vi "VALEW_ATC_Non-concurrent Verify Valve Timing.vi"(0 "High Times (s)":dbl[][](array[numeric])=[[0.048, 19.932000000000002, 0.0], [0.256, 9.626, 10.098], [0.254, 9.628, 10.098], [0.256, 9.625, 10.099], [0.047, 19.933, 0.0], [0.253, 10.701, 9.026], [0.255, 10.699, 9.026], [0.048, 19.932000000000002, 0.0], [0.258, 8.014, 11.708], [0.256, 8.016, 11.708], [0.256, 8.016, 11.708], [0.048, 19.932000000000002, 0.0], [0.254, 7.527, 12.199], [0.047, 19.933, 0.0], [0.253, 6.848, 12.879]], 7 "Total cold ON time (s)":dbl, 11 "Total hot ON time (s)":dbl) -> (6 "Pass/Fail?":bool, 10 "Report Text":string)   [LabVIEW 2016, in "TLMB.lvlib"]
uses:
  Projects/TLMB.lvlib
panel:
  # "off"
  # "on"
  # "off"
  # "on"
  # "off"
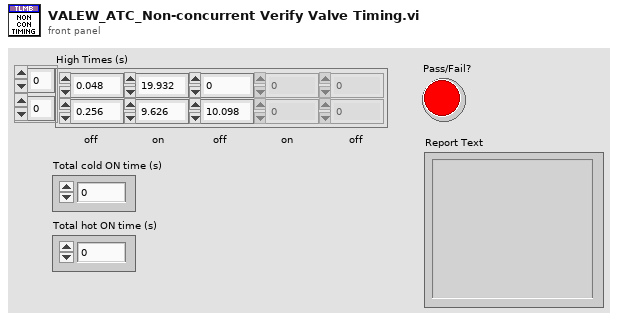
[diagram p1: front panel]
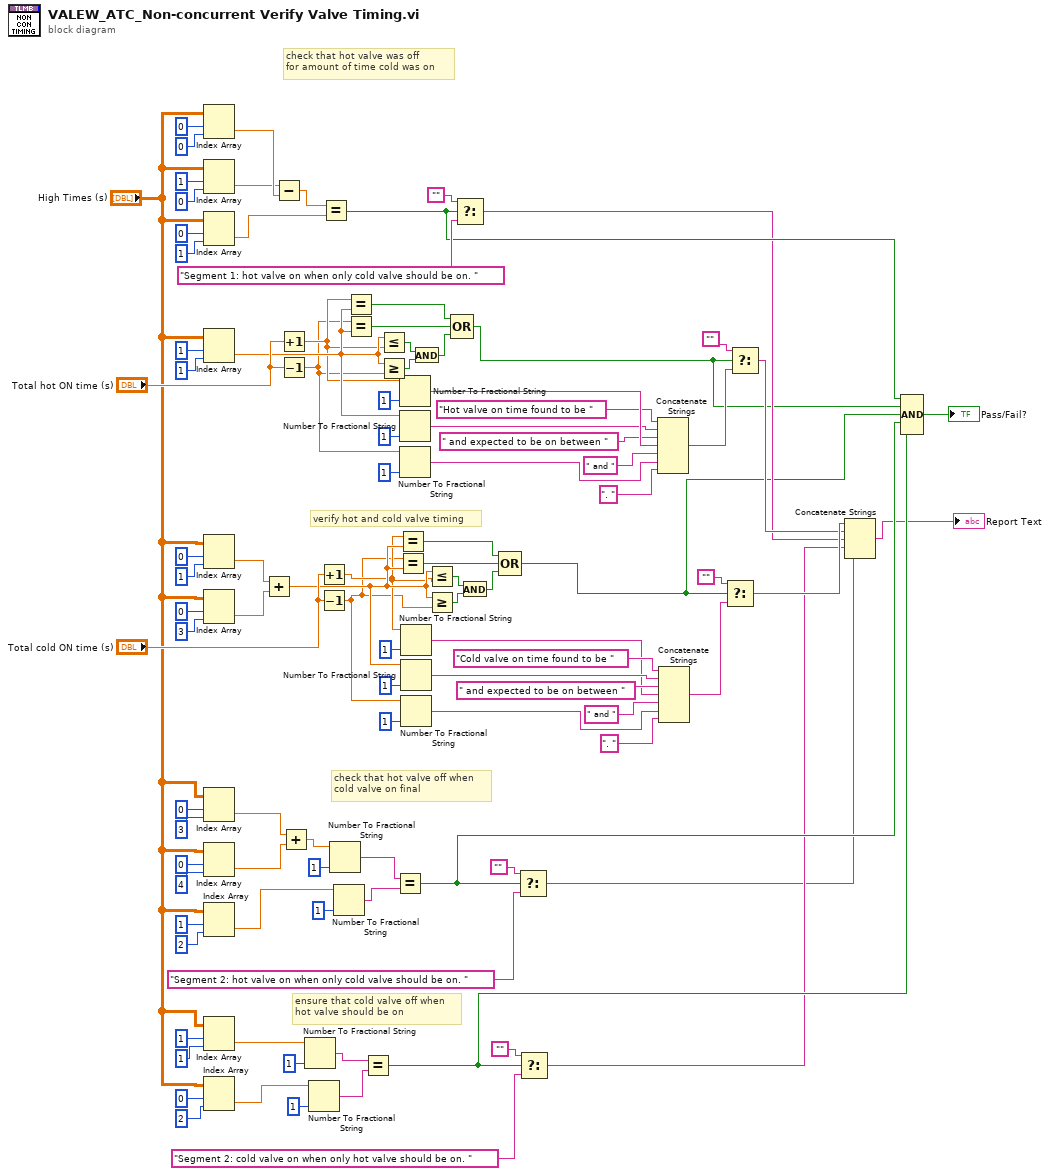
[diagram p0: block diagram]
diagram:
  # "verify hot and cold valve timing"
  # "ensure that cold valve off when\nhot valve should be on"
  # "check that hot valve off when\ncold valve on final"
  # "check that hot valve was off\nfor amount of time cold was on"
  n1 = Index Array(array="High Times (s)", index (row)=0, index (col)=0 ("disabled index (col)")) -> (element=w34:dbl)
  n2 = Index Array(array="High Times (s)", index (row)=1, index (col)=0 ("disabled index (col)")) -> (element=w33:dbl)
  n3 = Index Array(array="High Times (s)", index (row)=0, index (col)=1 ("disabled index (col)")) -> (element=w99:dbl)
  n4 = Index Array(array="High Times (s)", index (row)=1, index (col)=1 ("disabled index (col)")) -> (element=w15:dbl)
  n5 = Index Array(array="High Times (s)", index (row)=0, index (col)=1 ("disabled index (col)")) -> (element=w88:dbl)
  n6 = Index Array(array="High Times (s)", index (row)=0, index (col)=3 ("disabled index (col)")) -> (element=w89:dbl)
  n7 = Index Array(array="High Times (s)", index (row)=0, index (col)=3 ("disabled index (col)")) -> (element=w80:dbl)
  n8 = Index Array(array="High Times (s)", index (row)=0, index (col)=4 ("disabled index (col)")) -> (element=w79:dbl)
  n9 = Index Array(array="High Times (s)", index (row)=1, index (col)=2 ("disabled index (col)")) -> (element=w7:dbl)
  n10 = Index Array(array="High Times (s)", index (row)=1, index (col)=1 ("disabled index (col)")) -> (element=w1:dbl)
  n11 = Index Array(array="High Times (s)", index (row)=0, index (col)=2 ("disabled index (col)")) -> (element=w2:dbl)
  n12 = Add(x=w88, y=w89) -> (x+y=w21:dbl)
  n13 = Subtract(x=w33, y=w34) -> (x-y=w32:dbl)
  n14 = Increment(x="Total hot ON time (s)") -> (x+1=w14:dbl)
  n15 = Decrement(x="Total hot ON time (s)") -> (x-1=w13:dbl)
  n16 = Add(x=w80, y=w79) -> (x+y=w9:dbl)
  n17 = Number To Fractional String(number=w1, precision (6)=i16 1) -> (F-format string=w4:string)  [unwired: 2 in]
  n18 = Number To Fractional String(number=w2, precision (6)=i16 1) -> (F-format string=w3:string)  [unwired: 2 in]
  n19 = Increment(x="Total cold ON time (s)") -> (x+1=w20:dbl)
  n20 = Decrement(x="Total cold ON time (s)") -> (x-1=w19:dbl)
  n21 = Equal?(x=w32, y=w99) -> (x = y?=w46:bool)
  n22 = Number To Fractional String(number=w9, precision (6)=i16 1) -> (F-format string=w8:string)  [unwired: 2 in]
  n23 = Number To Fractional String(number=w7, precision (6)=i16 1) -> (F-format string=w11:string)  [unwired: 2 in]
  n24 = Equal?(x=w14, y=w15) -> (x = y?=w27:bool)
  n25 = Equal?(x=w13, y=w15) -> (x = y?=w26:bool)
  n26 = Equal?(x=w4, y=w3) -> (x = y?=w43:bool)
  n27 = Less Or Equal?(x=w15, y=w14) -> (x <= y?=w18:bool)
  n28 = Greater Or Equal?(x=w15, y=w13) -> (x >= y?=w17:bool)
  n29 = Equal?(x=w8, y=w11) -> (x = y?=w44:bool)
  n30 = Equal?(x=w20, y=w21) -> (x = y?=w29:bool)
  n31 = Equal?(x=w19, y=w21) -> (x = y?=w28:bool)
  n32 = Number To Fractional String(number=w14, precision (6)=i16 1) -> (F-format string=w68:string)  [unwired: 2 in]
  n33 = Number To Fractional String(number=w15, precision (6)=i16 1) -> (F-format string=w66:string)  [unwired: 2 in]
  n34 = Number To Fractional String(number=w13, precision (6)=i16 1) -> (F-format string=w70:string)  [unwired: 2 in]
  n35 = Number To Fractional String(number=w20, precision (6)=i16 1) -> (F-format string=w52:string)  [unwired: 2 in]
  n36 = Number To Fractional String(number=w21, precision (6)=i16 1) -> (F-format string=w54:string)  [unwired: 2 in]
  n37 = Number To Fractional String(number=w19, precision (6)=i16 1) -> (F-format string=w50:string)  [unwired: 2 in]
  n38 = And(x=w18, y=w17) -> (x .and. y?=w16:bool)
  n39 = Less Or Equal?(x=w21, y=w20) -> (x <= y?=w24:bool)
  n40 = Greater Or Equal?(x=w21, y=w19) -> (x >= y?=w23:bool)
  n41 = Compound Arithmetic op=OR(w27, w26, w16) -> (w25:bool)
  n42 = Select(t="", s=w46, f="Segment 1: hot valve on when only cold valve should be on. ") -> (s? t:f=w40:string)
  n43 = And(x=w24, y=w23) -> (x .and. y?=w22:bool)
  n44 = Compound Arithmetic op=OR(w29, w28, w22) -> (w30:bool)
  n45 = Select(t="", s=w44, f="Segment 2: hot valve on when only cold valve should be on. ") -> (s? t:f=w38:string)
  n46 = Select(t="", s=w43, f="Segment 2: cold valve on when only hot valve should be on. ") -> (s? t:f=w39:string)
  n47 = Concatenate Strings("Hot valve on time found to be ", w66, " and expected to be on between ", w68, " and " ("string"), w70, ". " ("string")) -> (w60:string)
  n48 = Concatenate Strings("Cold valve on time found to be ", w54, " and expected to be on between ", w52, " and " ("string"), w50, ". " ("string")) -> (w49:string)
  n49 = Select(t="", s=w30, f=w49) -> (s? t:f=w42:string)
  n50 = Select(t="", s=w25, f=w60) -> (s? t:f=w41:string)
  n51 = Concatenate Strings(w42, w41, w40, w39, w38) -> (→"Report Text":string)
  n52 = Compound Arithmetic op=AND(w46, w25, w30, w44, w43) -> (→"Pass/Fail?":bool)
